vi "Auto Variables.vi"() -> ()   [LabVIEW 2020]
panel:
  out "Time to Drive Forward":dbl
  out "Actual Distance Travelled":dbl
  out "Distance to Travel":dbl
  out "Start Delay (in Seconds)":dbl
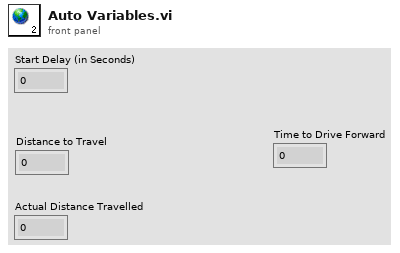
[diagram p1: front panel]
diagram:
